vi "CSU22 Parse Disk Speed.vi"(0 "Reply String":string, 11 "Error In":errorcluster) -> (8 "Speed (RPM)":i32, 15 "Error Out":errorcluster)   [LabVIEW 2020]
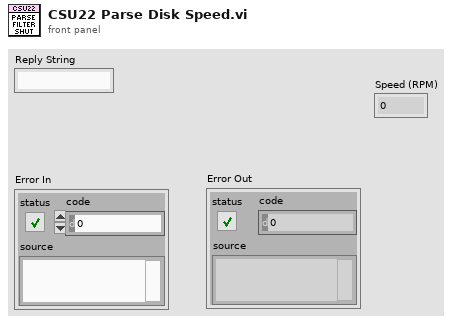
[diagram p1: front panel]
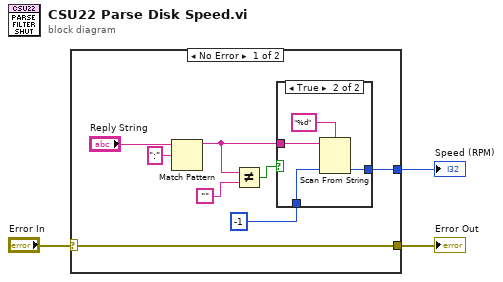
[diagram p0: block diagram]
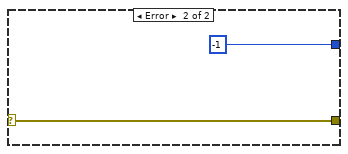
[diagram p3: hidden frame]
diagram:
  n1 = case shown="No Error" "Error In" {
    selector: "Error In" -> [w6 w18]
    tunnel: [w6 w18] -> w2
    tunnel: [w4 -1] -> w1
    frame No Error {
      n2 = Match Pattern(string="Reply String", regular expression=":") -> (before substring=w10:string)  [unwired: 1 in, 3 out]
      n3 = Not Equal?(x=w10, y="") -> (x != y?=w8:bool)
      n4 = case shown="True" w8 {
        tunnel: w10 -> [_ w16]
        tunnel: -1 -> [w12 w15]
        tunnel: [w12 w13] -> w4
        frame False {
        }
        frame True {
          n5 = Scan From String(format string="%d", input string=w16, default 1=w15) -> (output 1=w13:i32)  [unwired: 2 in, 3 out]
        }
      }
    }
    frame Error {
    }
  }
  "Error Out" <- w2
  "Speed (RPM)" <- w1
